vi "obtain_fit_parameters.vi"(7 "increment step":dbl[unit]=0.017453292519943295, 8 "error in (no error)":errorcluster, 10 "PointCollection B":refnum<class "PointCollection.lvclass">, 11 "PointCollection in":refnum<class "PointCollection.lvclass">) -> (0 "error out":errorcluster, 1 "scale factor":dbl, 2 "translation vector":dbl[](array[numeric]), 3 "PointCollection out":refnum<class "PointCollection.lvclass">, 4 "rotation fit angles":dbl[unit][](array[numeric]))   [LabVIEW 2010, in "PointCollection.lvclass"]
uses:
  PointCollection.lvclass
  mode_enum.ctl
  x_y_z_enumeration.ctl
  <vilib>/Analysis/NI_AALBase.lvlib
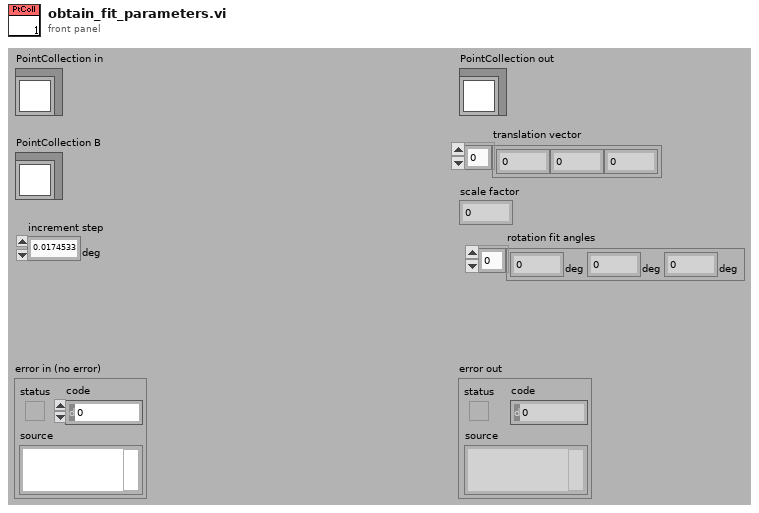
[diagram p1: front panel]
types:
  T1 = typedef "PointCollection.lvclass/x_y_z_enumeration.ctl" = enum16{"x", "y", "z"}
  T2 = typedef "PointCollection.lvclass/mode_enum.ctl" = enum16{"points first", "dimensions first"}
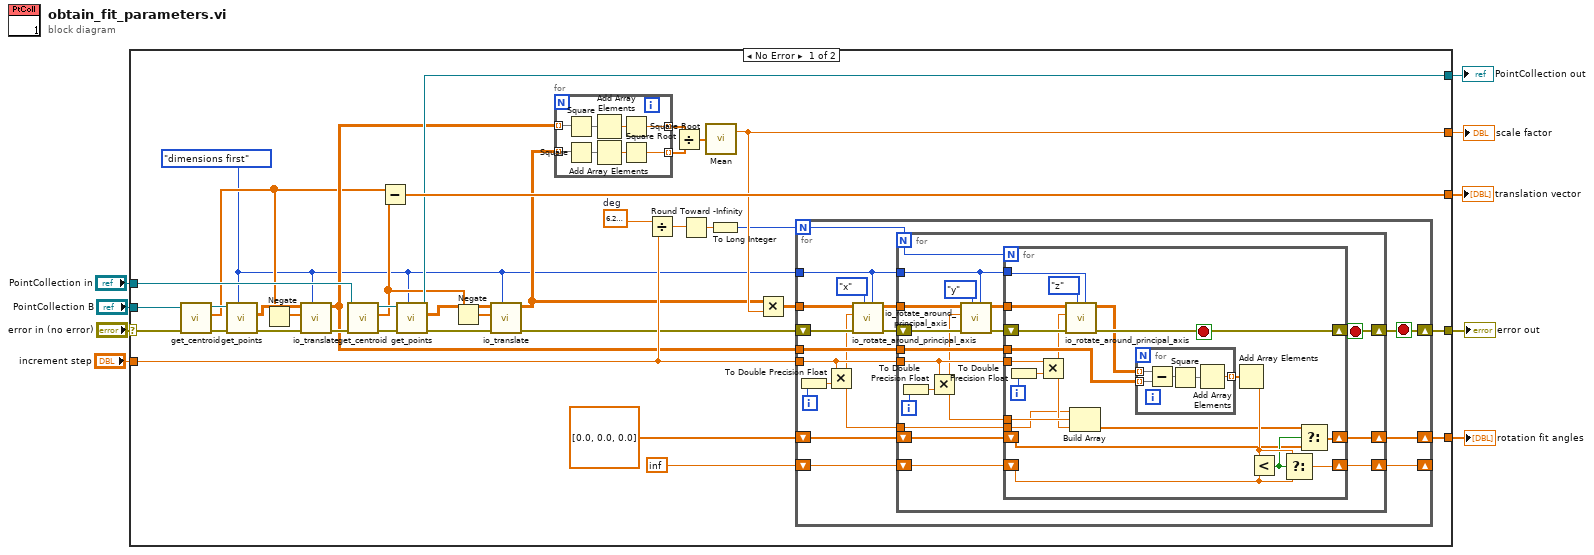
[diagram p0: block diagram]
diagram:
  n1 = case shown="No Error" "error in (no error)" {
    selector: "error in (no error)" -> [w44 w116]
    tunnel: [w34 w116] -> w8
    tunnel: [w31 w115] -> w6
    tunnel: "PointCollection in" -> [w43 w115]
    tunnel: "PointCollection B" -> [w45 _]
    tunnel: [w42 _] -> w4
    tunnel: [w33 _] -> w3
    tunnel: "increment step" -> [w29 _]
    tunnel: [w24 _] -> w1
    frame No Error {
      w10 = mode_enum."dimensions first" ("retrieval mode")
      w30 = dbl[unit] 6.283185307179586  # deg
      n2 = call-dynamic "get_centroid.vi"("error in (no error)"=w44, "PointCollection in"=w45) -> ("error out"=w39:errorcluster, "centroid"=w18:dbl[], "PointCollection out"=w38:refnum<class "PointCollection.lvclass">)  [unwired: 7 in]
      n3 = call-dynamic "get_points.vi"("retrieval mode"=w10, "error in (no error)"=w39, "PointCollection in"=w38) -> ("error out"=w22:errorcluster, "points"=w20:dbl[][])  [unwired: 6 in, 1 out]
      n4 = Negate(x=w18) -> (-x=w13:dbl[])
      n5 = call "io_translate.vi"("mode"=w10, "error in (no error)"=w22, "vector"=w13, "points in"=w20) -> ("error out"=w21:errorcluster, "points out"=w19:dbl[][])  [unwired: 6 in]
      n6 = call-dynamic "get_centroid.vi"("error in (no error)"=w21, "PointCollection in"=w43) -> ("error out"=w41:errorcluster, "centroid"=w12:dbl[], "PointCollection out"=w40:refnum<class "PointCollection.lvclass">)  [unwired: 7 in]
      n7 = Subtract(x=w18, y=w12) -> (x-y=w42:dbl[])
      n8 = call-dynamic "get_points.vi"("retrieval mode"=w10, "error in (no error)"=w41, "PointCollection in"=w40) -> ("error out"=w17:errorcluster, "points"=w15:dbl[][], "PointCollection out"=w31:refnum<class "PointCollection.lvclass">)  [unwired: 6 in]
      n9 = Negate(x=w12) -> (-x=w11:dbl[])
      n10 = call "io_translate.vi"("mode"=w10, "error in (no error)"=w17, "vector"=w11, "points in"=w15) -> ("error out"=w16:errorcluster, "points out"=w14:dbl[][])  [unwired: 6 in]
      n11 = for {
        tunnel: w19 -> [w112] mode=indexing
        tunnel: w14 -> [w109] mode=indexing
        tunnel: [w108] -> w37 mode=indexing
        tunnel: [w107] -> w36 mode=indexing
        n12 = Square(x=w112) -> (x^2=w114:dbl[])
        n13 = Square(x=w109) -> (x^2=w110:dbl[])
        n14 = Add Array Elements(numeric array=w114) -> (sum=w113:dbl)
        n15 = Add Array Elements(numeric array=w110) -> (sum=w111:dbl)
        n16 = Square Root(x=w113) -> (sqrt(x)=w108:dbl)
        n17 = Square Root(x=w111) -> (sqrt(x)=w107:dbl)
      }
      n18 = Divide(x=w30, y=w29) -> (x/y=w28:dbl)
      n19 = Divide(x=w37, y=w36) -> (x/y=w35:dbl[])
      n20 = Round Toward -Infinity(1:w28) -> (0:w27:dbl)
      n21 = call <vilib>:"Mean.vi"("X"=w35) -> ("mean"=w33:dbl)  [unwired: 1 out]
      n22 = To Long Integer(number=w27) -> (32bit integer=w26:i32)
      n23 = Multiply(x=w14, y=w33) -> (x*y=w32:dbl[][])
      n24 = for {
        N: w26 -> [w52]
        tunnel: w32 -> [w58]
        tunnel: w19 -> [w62]
        shift-right: [w61] -> w34
        shift-left: w16 -> [w60]
        tunnel: w29 -> [w55]
        shift-right: [w50] -> w24
        shift-left: dbl[unit][] [0.0, 0.0, 0.0] ("rotation fit angles") -> [w51]
        shift-right: [w48] -> _
        shift-left: inf -> [w49]
        tunnel: w10 -> [w46]
        i -> [w56]
        stop <- w61 stop-if-true
        n25 = To Double Precision Float(number=w56) -> (double precision float=w53:dbl)
        n26 = Multiply(x=w55, y=w53) -> (x*y=w47:dbl[unit])
        n27 = call "io_rotate_around_principal_axis.vi"("mode"=w46, "axis"=x_y_z_enumeration."x", "error in (no error)"=w60, "angle"=w47, "points in"=w58) -> ("error out"=w59:errorcluster, "points out"=w57:dbl[][])  [unwired: 5 in]
        n28 = for {
          N: w52 -> [w71]
          tunnel: w62 -> [w80]
          tunnel: w57 -> [w77]
          tunnel: w55 -> [w73]
          shift-right: [w70] -> w61
          shift-left: w59 -> [w79]
          shift-right: [w68] -> w50
          shift-left: w51 -> [w69]
          shift-right: [w66] -> w48
          shift-left: w49 -> [w67]
          tunnel: w47 -> [w64]
          tunnel: w46 -> [w63]
          i -> [w75]
          stop <- w70 stop-if-true
          n29 = To Double Precision Float(number=w75) -> (double precision float=w74:dbl)
          n30 = Multiply(x=w73, y=w74) -> (x*y=w65:dbl[unit])
          n31 = call "io_rotate_around_principal_axis.vi"("mode"=w63, "axis"=x_y_z_enumeration."y", "error in (no error)"=w79, "angle"=w65, "points in"=w77) -> ("error out"=w78:errorcluster, "points out"=w76:dbl[][])  [unwired: 5 in]
          n32 = for {
            N: w71 -> [_]
            shift-right: [w99] -> w70
            shift-left: w78 -> [w101]
            tunnel: w80 -> [w93]
            tunnel: w73 -> [w97]
            tunnel: w76 -> [w98]
            shift-right: [w87] -> w68
            shift-left: w69 -> [w86]
            shift-right: [w90] -> w66
            shift-left: w67 -> [w91]
            tunnel: w65 -> [w85]
            tunnel: w64 -> [w82]
            tunnel: w63 -> [w81]
            i -> [w96]
            stop <- w99 stop-if-true
            n33 = To Double Precision Float(number=w96) -> (double precision float=w95:dbl)
            n34 = Multiply(x=w97, y=w95) -> (x*y=w83:dbl[unit])
            n35 = call "io_rotate_around_principal_axis.vi"("mode"=w81, "axis"=x_y_z_enumeration."z", "error in (no error)"=w101, "angle"=w83, "points in"=w98) -> ("error out"=w99:errorcluster, "points out"=w94:dbl[][])  [unwired: 5 in]
            n36 = Build Array(w82, w85, w83) -> (w84:dbl[unit][])
            n37 = for {
              tunnel: w94 -> [w106] mode=indexing
              tunnel: w93 -> [w105] mode=indexing
              tunnel: [w102] -> w92 mode=indexing
              n38 = Subtract(x=w106, y=w105) -> (x-y=w104:dbl[])
              n39 = Square(x=w104) -> (x^2=w103:dbl[])
              n40 = Add Array Elements(numeric array=w103) -> (sum=w102:dbl)
            }
            n41 = Add Array Elements(numeric array=w92) -> (sum=w89:dbl)
            n42 = Less?(x=w89, y=w91) -> (x < y?=w88:bool)
            n43 = Select(t=w89, s=w88, f=w91) -> (s? t:f=w90:dbl)
            n44 = Select(t=w84, s=w88, f=w86) -> (s? t:f=w87:dbl[unit][])
          }
        }
      }
    }
    frame Error {
    }
  }
  "error out" <- w8
  "PointCollection out" <- w6
  "scale factor" <- w3
  "translation vector" <- w4
  "rotation fit angles" <- w1
